vi "SendVLCCommand.vi"(8 "error in":errorcluster, 9 "Argument":string, 10 "Command":T1, 11 "Connection ID in":refnum<k5>) -> (0 "error out":errorcluster, 1 "bytes written":i32, 2 "Messages":string, 3 "Connection ID out":refnum<k5>)   [LabVIEW 2015]
doc: "Send a command to the VLC instance. Some of the commands require an argument, which can be provided as a string. Others do not, and the argument input can be left as the default, an empty string.\n\nThe following is a copy of the command documentation help provided by the VLC RC interface:\n\n+----[ Remote control commands ]\n|\n| add XYZ . . . . . . . . . . . . add XYZ to playlist\n| enqueue XYZ . . . . . . . . . queue XYZ to playlist\n| playlist . . . . . show items currently in playlist\n| play . . . . . . . . . . . . . . . . . . play stream\n| stop . . . . . . . . . . . . . . . . . . stop stream\n| next . . . . . . . . . . . . . . next playlist item\n| prev . . . . . . . . . . . . previous playlist item\n| goto . . . . . . . . . . . . . . goto item at index\n| repeat [on|off] . . . . toggle playlist item repeat\n| loop [on|off] . . . . . . . . . toggle playlist loop\n| random [on|off] . . . . . . . toggle random jumping\n| clear . . . . . . . . . . . . . . clear the playlist\n| status . . . . . . . . . . . current playlist status\n| title [X] . . . . . . set/get title in current item\n| title_n . . . . . . . . next title in current item\n| title_p . . . . . . previous title in current item\n| chapter [X] . . . . set/get chapter in current item\n| chapter_n . . . . . . next chapter in current item\n| chapter_p . . . . previous chapter in current item\n|\n| seek X . . . seek in seconds, for instance `seek 12'\n| pause . . . . . . . . . . . . . . . . toggle pause\n| fastforward . . . . . . . . . set to maximum rate\n| rewind . . . . . . . . . . . . set to minimum rate\n| faster . . . . . . . . . . faster playing of stream\n| slower . . . . . . . . . . slower playing of stream\n| normal . . . . . . . . . . normal playing of stream\n| frame. . . . . . . . . . play frame by frame\n| f [on|off] . . . . . . . . . . . . toggle fullscreen\n| info . . . . . information about the current stream\n| stats . . . . . . . . show statistical information\n| get_time . . seconds elapsed since stream's beginning\n| is_playing . . . . 1 if a stream plays, 0 otherwise\n| get_title . . . . . the title of the current stream\n| get_length . . . . the length of the current stream\n|\n| volume [X] . . . . . . . . . . set/get audio volume\n| volup [X] . . . . . . . raise audio volume X steps\n| voldown [X] . . . . . . lower audio volume X steps\n| adev [device] . . . . . . . . set/get audio device\n| achan [X]. . . . . . . . . . set/get audio channels\n| atrack [X] . . . . . . . . . . . set/get audio track\n| vtrack [X] . . . . . . . . . . . set/get video track\n| vratio [X] . . . . . . . set/get video aspect ratio\n| vcrop [X] . . . . . . . . . . . set/get video crop\n| vzoom [X] . . . . . . . . . . . set/get video zoom\n| snapshot . . . . . . . . . . . . take video snapshot\n| strack [X] . . . . . . . . . set/get subtitle track\n| key [hotkey name] . . . . . . simulate hotkey press\n|\n| help . . . . . . . . . . . . . . . this help message\n| logout . . . . . . . exit (if in socket connection)\n| quit . . . . . . . . . . . . . . . . . . . quit vlc\n|\n+----[ end of help ]"
uses:
  VLCCommand.ctl
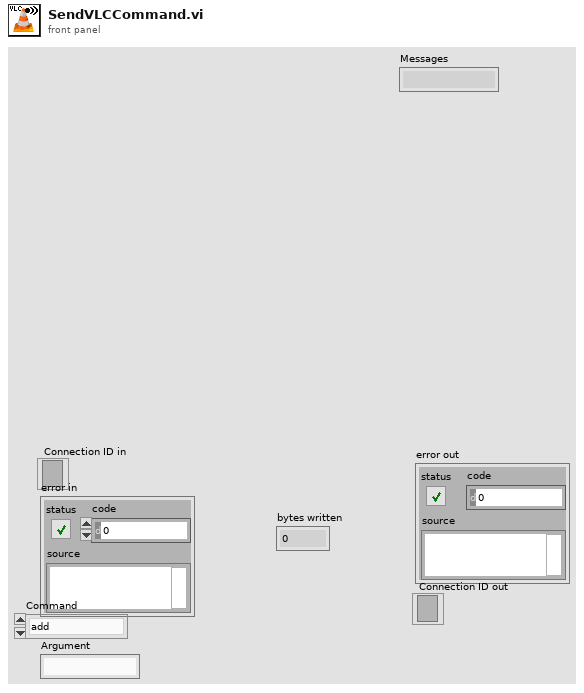
[diagram p1: front panel]
types:
  T1 = typedef "VLCCommand.ctl" = enum16{"add", "enqueue", "playlist", "play", "stop", "next", "prev", "goto", "repeat", "loop", "random", "clear", "status", "title", "title_n", "title_p", "chapter", "chapter_n", "chapter_p", "seek", "pause", "fastforward", "rewind", "faster", "slower", "normal", "frame", "f", "info", "stats", "get_time", "is_playing", "get_title", "get_length", "volume", "volup", "voldown", "adev", "achan", "atrack", "vtrack", "vratio", "vcrop", "vzoom", "snapshot", "strack", "key", "help", "logout", "quit"}
  T2 = enum16{"Standard", "Buffered", "CRLF", "Immediate"}
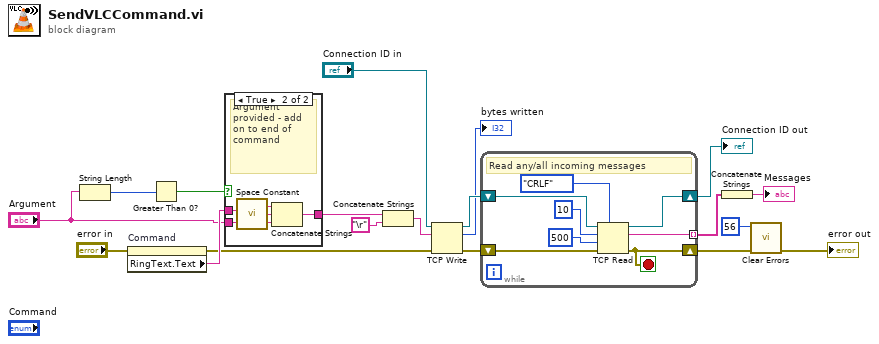
[diagram p0: block diagram]
diagram:
  n1 = String Length(string="Argument") -> (length=w14:i32)
  n2 = property on="Command" class="Enum (strict)"(error in="error in") -> (error out=w8:errorcluster, "RingText.Text"=w12:string)  [unwired: 1 in, 1 out]
  n3 = Greater Than 0?(x=w14) -> (x > 0?=w13:bool)
  n4 = case shown="True" w13 {
    tunnel: w12 -> [w20 w23]
    tunnel: "Argument" -> [_ w22]
    tunnel: [w20 w21] -> w10
    frame False {
      # "No argument provided"
    }
    frame True {
      # "Argument provided - add on to end of command"
      n5 = call <vilib>:"Space Constant.vi"() -> ("String"=w24:string)
      n6 = Concatenate Strings(w23, w24, w22) -> (w21:string)
    }
  }
  n7 = Concatenate Strings(w10, "\r") -> (w17:string)
  n8 = TCP Write(connection ID="Connection ID in", data in=w17, error in (no error)=w8) -> (connection ID out=w19:refnum<k5>, bytes written=→"bytes written":i32, error out=w7:errorcluster)  [unwired: 1 in]
  n9 = while {
    shift-right: [w31] -> w15
    shift-left: w19 -> [w32]
    tunnel: [w28] -> w5 mode=indexing
    shift-right: [w25] -> w6
    shift-left: w7 -> [w26]
    stop <- w25 stop-if-true
    # "Read any/all incoming messages"
    n10 = TCP Read(connection ID=w32, bytes to read=10, error in (no error)=w26, 7:T2."CRLF" ("mode (standard)"), 9:500 ("timeout ms (25000)")) -> (connection ID out=w31:refnum<k5>, data out=w28:string, error out=w25:errorcluster)
  }
  "Connection ID out" <- w15
  n11 = Concatenate Strings(w5) -> (→"Messages":string)
  n12 = call <vilib>:"Clear Errors.vi"("error in (no error)"=w6, "specific error code to clear (0: all)"=56) -> ("error out"=→"error out":errorcluster)  [unwired: 4 in, 1 out]
